vi "odometry.vi"(7 "ENCB in":dbl, 8 "ENCA in":dbl, 9 "wheelbase":dbl=250.0, 10 "Position":T1) -> (0 "ENCB OUT":i32, 1 "ENCA OUT":i32, 3 "X, Y, BEARING":cluster{dbl, dbl, dbl})   [LabVIEW 2017]
uses:
  040-typeDefs/Position.ctl
  <vilib>/myRIO/Common/Instrument Driver Framework/myRIO v1.0/Encoder/typedefs/Encoder Signal Mode.ctl
  <vilib>/myRIO/Instrument Drivers/Onboard IO/Encoder/typedefs/Encoder Reference.ctl
  <vilib>/myRIO/Common/Instrument Driver Framework/Utilities/typedefs/myRIO Generic Hardware Reference.ctl
  <vilib>/myRIO/Common/Instrument Driver Framework/Utilities/typedefs/Hardware Version Enum.ctl
  <vilib>/myRIO/Common/Instrument Driver Framework/Utilities/typedefs/myRIO v1.0 Reference.ctl
  <vilib>/myRIO/Common/Instrument Driver Framework/Utilities/typedefs/Generic FPGA Reference.ctl
  <vilib>/myRIO/Common/Instrument Driver Framework/myRIO v1.0/Encoder/typedefs/Encoder Channels Enum.ctl
  <vilib>/myRIO/Common/Instrument Driver Framework/myRIO v1.0/Encoder/typedefs/Encoder Configuration v1.0.ctl
  <vilib>/userdefined/High Color/nirio_resource_hc.ctl
  <vilib>/myRIO/Common/Instrument Driver Framework/Utilities/vis/Is FPGA Ref Available.vi
  <vilib>/myRIO/Common/Instrument Driver Framework/myRIO v1.0/Encoder/vis/myRIO v1.1 Open Encoder.vi
  <vilib>/myRIO/Instrument Drivers/Onboard IO/Encoder/vis/Read.vi
  <vilib>/myRIO/Common/Instrument Driver Framework/Utilities/vis/Validate Channels.vi
  <vilib>/myRIO/Common/Instrument Driver Framework/myRIO v1.0/Encoder/vis/myRIO v1.0 Reserve Encoder.vi
  <vilib>/myRIO/Common/Instrument Driver Framework/myRIO v1.0/Encoder/vis/myRIO v1.0 Build MUX Configuration Encoder.vi
  <vilib>/myRIO/Common/Instrument Driver Framework/myRIO v1.0/Resource Manager/vis/myRIO v1.0 Reserve Channel List.vi
  <vilib>/myRIO/Common/Instrument Driver Framework/myRIO v1.0/Resource Manager/vis/myRIO v1.0 Create Configuration List.vi
  <vilib>/myRIO/Common/Instrument Driver Framework/myRIO v1.0/Resource Manager/vis/myRIO v1.0 Reserve Channel.vi
  <vilib>/myRIO/Common/Instrument Driver Framework/myRIO v1.0/Resource Manager/vis/myRIO v1.0 Unreserve Channel.vi
  <vilib>/myRIO/Common/Instrument Driver Framework/myRIO v1.0/Resource Manager/vis/myRIO v1.0 Build Mutex Name.vi
  <vilib>/Utility/VariantDataType/GetNumericInfo.vi
  <vilib>/Utility/error.llb/Error Cluster From Error Code.vi
  <vilib>/myRIO/Common/Instrument Driver Framework/myRIO v1.0/myRIO v1.1 Open.vi
  <vilib>/myRIO/Common/Instrument Driver Framework/Utilities/vis/IO Manager.vi
  <vilib>/myRIO/Common/Instrument Driver Framework/Utilities/vis/Configuration Manager.vi
  <vilib>/myRIO/Common/Instrument Driver Framework/myRIO v1.0/Resource Manager/vis/myRIO v1.0 Configure IO.vi
  <vilib>/myRIO/Common/Instrument Driver Framework/myRIO v1.0/myRIO v1.0 Close.vi
  <vilib>/myRIO/Common/Instrument Driver Framework/myRIO v1.0/Encoder/vis/myRIO v1.0 Configure Encoder.vi
  <vilib>/myRIO/Common/Instrument Driver Framework/myRIO v1.0/Encoder/vis/myRIO v1.0 Read Encoder.vi
  <vilib>/myRIO/Express VI/Onboard IO/Encoder/Encoder Express VI.xnode
  <vilib>/myRIO/Instrument Drivers/Onboard IO/Encoder/vis/myRIO Encoder Open.xnode
  <vilib>/myRIO/Instrument Drivers/Onboard IO/Encoder/Encoder.lvlib
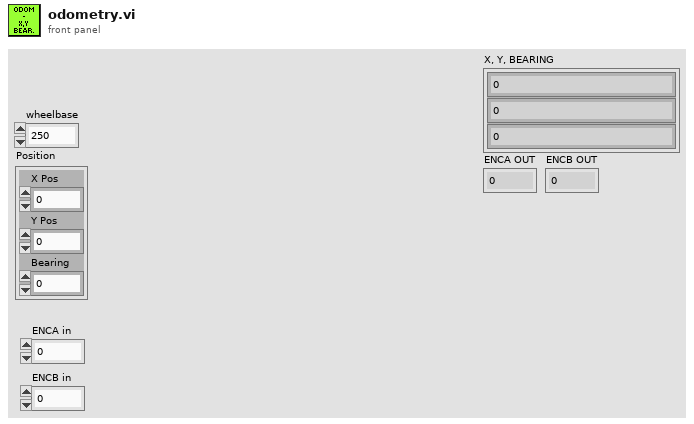
[diagram p1: front panel]
types:
  T1 = typedef "Position.ctl" = cluster{"X Pos":dbl, "Y Pos":dbl, "Bearing":dbl}
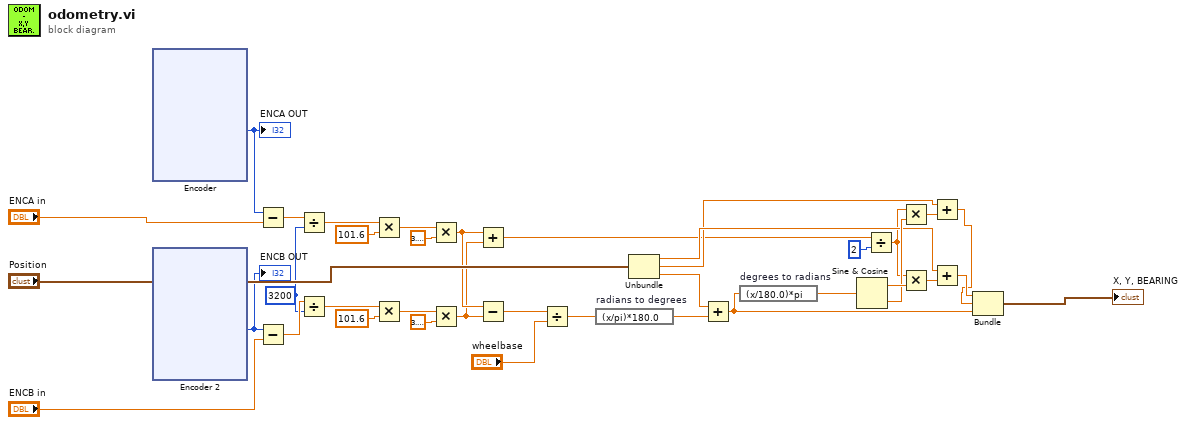
[diagram p0: block diagram]
diagram:
  w13 = 3200
  n1 = xnode "Encoder"() -> ("Counter Value"=w21:i32)  [unwired: 2 in, 3 out]
  "ENCA OUT" <- w21
  n2 = xnode "Encoder 2"() -> ("Counter Value"=w18:i32)  [unwired: 2 in, 3 out]
  "ENCB OUT" <- w18
  n3 = Subtract(x=w21, y="ENCA in") -> (x-y=w15:dbl)
  n4 = Subtract(x=w18, y="ENCB in") -> (x-y=w14:dbl)
  n5 = Divide(x=w15, y=w13) -> (x/y=w12:dbl)
  n6 = Divide(x=w14, y=w13) -> (x/y=w4:dbl)
  n7 = Multiply(x=w12, y=101.6) -> (x*y=w11:dbl)
  n8 = Multiply(x=w4, y=101.6) -> (x*y=w6:dbl)
  n9 = Multiply(x=w11, y=3.141592653589793) -> (x*y=w10:dbl)
  n10 = Multiply(x=w6, y=3.141592653589793) -> (x*y=w5:dbl)
  n11 = Add(x=w10, y=w5) -> (x+y=w16:dbl)
  n12 = Subtract(x=w10, y=w5) -> (x-y=w17:dbl)
  n13 = Divide(x=w17, y="wheelbase") -> (x/y=w34:dbl)
  n14 = expression code="(x/pi)*180.0" "radians to degrees"(w34) -> (w32:dbl)
  n15 = Unbundle("Position") -> ("X Pos"=w25:dbl, "Y Pos"=w24:dbl, "Bearing"=w33:dbl)
  n16 = Add(x=w33, y=w32) -> (x+y=w31:dbl)
  n17 = expression code="(x/180.0)*pi" "degrees to radians"(w31) -> (w30:dbl)
  n18 = Sine & Cosine(0:w30) -> (1:w29:dbl, 2:w28:dbl)
  n19 = Divide(x=w16, y=2) -> (x/y=w22:dbl)
  n20 = Multiply(x=w22, y=w28) -> (x*y=w27:dbl)
  n21 = Multiply(x=w22, y=w29) -> (x*y=w26:dbl)
  n22 = Add(x=w24, y=w27) -> (x+y=w1:dbl)
  n23 = Add(x=w25, y=w26) -> (x+y=w2:dbl)
  n24 = Bundle(w2, w1, w31) -> (→"X, Y, BEARING":cluster{dbl, dbl, dbl})  [unwired: 1 in]
